vi "Actor Core.vi"(8 "error in":errorcluster, 11 "MC Prompt in":refnum<class "MC Prompt.lvclass">) -> (0 "error out":errorcluster, 3 "Actor out":refnum<class "Actor.lvclass">)   [LabVIEW 2024, in "MC Prompt.lvlib" / "MC Prompt.lvclass"]
doc: "<p>(<strong>Filename</strong>: <span class=\"dnl\">Actor Framework.lvlib:Actor.lvclass:Actor Core.vi</span>)</p>\n<p>Receives messages to the actor, reacts to them, and initiates any error handling that may shut the actor down.</p>\n<p>Descendant classes may override this VI to append parallel tasks for the actor to complete while it handles messages. Overrides use the <a href=\"nihelplauncher://docs/csh?context=lvcore_glang_udclass\">Call Parent Class Method</a> node.</p>"
uses:
  MC Prompt.lvclass
  C:/Program Files/National Instruments/LabVIEW 2024/vi.lib/ActorFramework/Actor/Actor.lvclass
  <vilib>/ActorFramework/Actor/Actor.lvclass
  MC Prompt.lvclass/MC Prompt.ctl
  <vilib>/ActorFramework/Actor/Actor.lvclass/Actor.ctl
  <vilib>/ActorFramework/Message Enqueuer/Message Enqueuer.lvclass/Message Enqueuer.ctl
  <vilib>/ActorFramework/Message Enqueuer/Init from Existing Queue.vi
  <vilib>/ActorFramework/Message Enqueuer/Enqueue.vi
  MC Prompt Messages/Correct Answer Msg/Correct Answer Msg.lvclass
  C:/Program Files/National Instruments/LabVIEW 2024/vi.lib/ActorFramework/Message/Message.lvclass
  MC Prompt Messages/Incorrect Answer Msg/Incorrect Answer Msg.lvclass
  <vilib>/ActorFramework/Stop Msg/Stop Msg.lvclass
  Controller/Controller Messages/Load Main Panel Display Msg/Load Main Panel Display Msg.lvclass
  Controller/Controller Messages/Reset Contestant Lights Msg/Reset Contestant Lights Msg.lvclass
  <vilib>/ActorFramework/Message Priority Queue/Priority Enqueue.vi
  <vilib>/ActorFramework/Message Enqueuer/Message Enqueuer.lvclass
panel:
  in  "Exit":bool
  out "Boolean 4":bool caption="555"
  out "Boolean 3":bool caption="dfsdf"
  out "Boolean 2":bool caption="asdfadfs"
  out "Boolean":bool caption="asdfasdf"
  out "Timer":dbl(slide)=44.0 scale=0.0..100.0
  in  "Correctly Answered":bool
  in  "Incorrect":bool
  out "Correct Answer":string="This is the answer you're looking for from the contestant"
  out "Question To Read Aloud":string="This is where the prompt to be read alout to the audience appears"
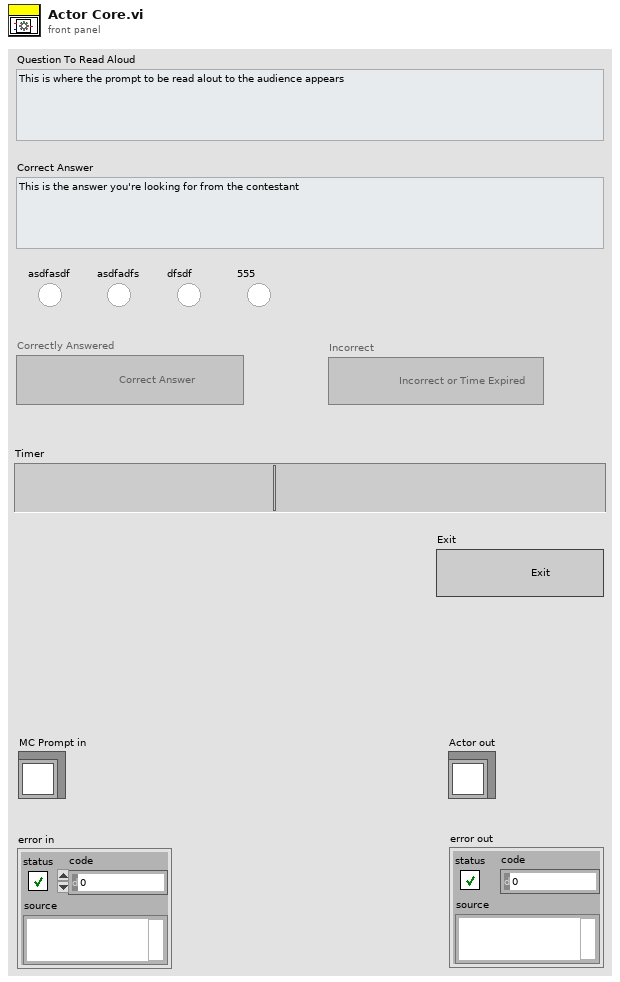
[diagram p1: front panel]
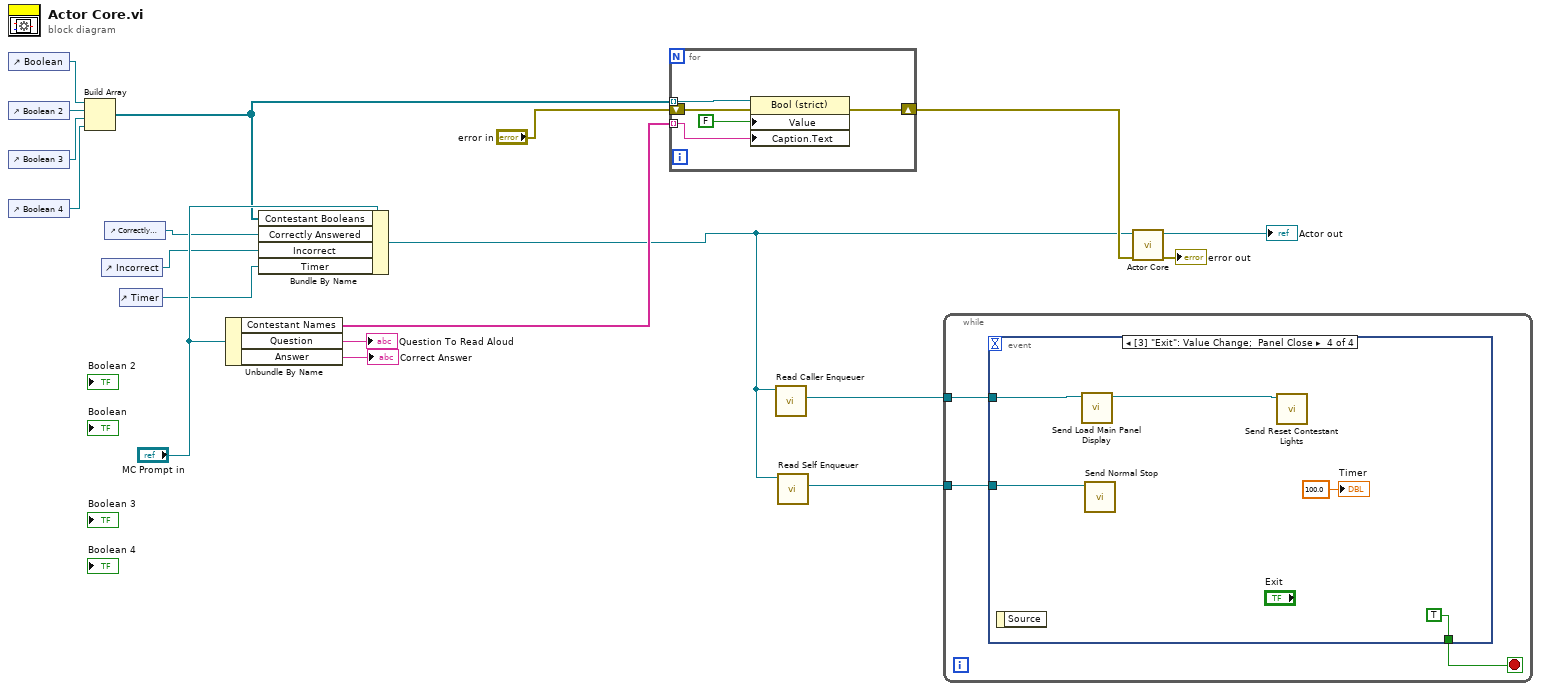
[diagram p0: block diagram]
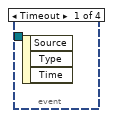
[diagram p2: hidden frame]
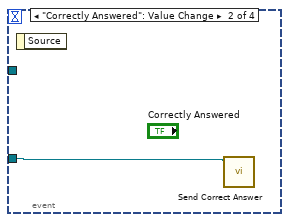
[diagram p3: hidden frame]
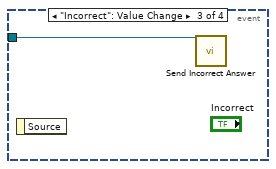
[diagram p4: hidden frame]
diagram:
  n1 = control-ref of="Boolean"() -> (w13:refnum<vi>)
  n2 = control-ref of="Boolean 2"() -> (w12:refnum<vi>)
  n3 = control-ref of="Boolean 3"() -> (w11:refnum<vi>)
  n4 = control-ref of="Boolean 4"() -> (w10:refnum<vi>)
  n5 = Build Array(w13, w12, w11, w10) -> (w14:refnum<vi>[])
  n6 = control-ref of="Incorrect"() -> (w5:refnum<vi>)
  n7 = control-ref of="Correctly Answered"() -> (w6:refnum<vi>)
  n8 = control-ref of="Timer"() -> (w1:refnum<vi>)
  n9 = Unbundle By Name("MC Prompt in") -> ("Contestant Names"=w9:string[], "Question"=→"Question To Read Aloud":string, "Answer"=→"Correct Answer":string)
  n10 = Bundle By Name(cluster="MC Prompt in", "Contestant Booleans"=w14, "Correctly Answered"=w6, "Incorrect"=w5, "Timer"=w1) -> (w3:refnum<class "MC Prompt.lvclass">)
  n11 = for {
    tunnel: w14 -> [w23] mode=indexing
    tunnel: w9 -> [w22] mode=indexing
    shift-right: [w21] -> w8
    shift-left: "error in" -> [w20]
    n12 = property class="Bool (strict)"(reference=w23, error in=w20, "Value"=FALSE, "Caption.Text"=w22) -> (error out=w21:errorcluster)  [unwired: 1 out]
  }
  n13 = call <vilib>:"Read Caller Enqueuer.vi"("Actor"=w3) -> ("Caller Enqueuer"=w4:refnum<class "Message Enqueuer.lvclass">)  [unwired: 10 in]
  n14 = call <vilib>:"Read Self Enqueuer.vi"("Actor"=w3) -> ("Self Enqueuer"=w2:refnum<class "Message Enqueuer.lvclass">)  [unwired: 10 in]
  n15 = while {
    tunnel: w4 -> [w27]
    tunnel: w2 -> [w25]
    stop <- w26 stop-if-true
    n16 = event shown="[3] \"Exit\": Value Change;  Panel Close" {
      selector: _ -> [_ _ _ _]
      dyn-events: _ -> [_ _ _ _]
      timeout: _ -> [_ _ _ _]
      tunnel: w27 -> [_ _ _ w33]
      tunnel: [_ _ _ TRUE] -> w26
      tunnel: w25 -> [_ w28 w29 w32]
      event Timeout {
        n17 = event-data() -> ()  [unwired: 1 in, 3 out]
      }
      event "Correctly Answered": Value Change {
        n18 = event-data() -> ()  [unwired: 1 in, 1 out]
        n19 = call "Send Correct Answer.vi"("Message Enqueuer"=w28) -> ()  [unwired: 9 in, 2 out]
      }
      event "Incorrect": Value Change {
        n20 = event-data() -> ()  [unwired: 1 in, 1 out]
        n21 = call "Send Incorrect Answer.vi"("Message Enqueuer"=w29) -> ()  [unwired: 9 in, 2 out]
      }
      event "Exit": Value Change; Panel Close {
        n22 = event-data() -> ()  [unwired: 1 in, 1 out]
        n23 = call "Send Load Main Panel Display.vi"("Message Enqueuer"=w33) -> ("Message Enqueuer out"=w31:refnum<class "Message Enqueuer.lvclass">)  [unwired: 9 in, 1 out]
        n24 = call <vilib>:"Send Normal Stop.vi"("Message Enqueuer"=w32) -> ()  [unwired: 10 in, 1 out]
        n25 = call "Send Reset Contestant Lights.vi"("Message Enqueuer"=w31) -> ()  [unwired: 9 in, 2 out]
        "Timer" <- 100.0 ("Timer")
      }
    }
  }
  n26 = call-parent "Actor Core.vi"("error in"=w8, "Actor in"=w3) -> ("error out"=→"error out":errorcluster, "Actor out"=→"Actor out":refnum<class "Actor.lvclass">)  [unwired: 8 in]
